vi "Main Page.vi"(8 "error in (no error)":errorcluster, 11 "Node Ptr":T1 format="%.0x") -> (0 "error out":errorcluster)   [LabVIEW 2012, in "PXImc System Explorer.lvlib"]
uses:
  PXImc System Explorer.lvlib
  <vilib>/NI Veristand/Custom Device API/Custom Device Item Ref.ctl
  Shared/Constants.vi
  <vilib>/NI Veristand/Custom Device API/Get Item Property (String).vi
  <vilib>/NI Veristand/Custom Device API/Get Item Property (U16).vi
  <vilib>/NI Veristand/Custom Device API/Set Item Property (String).vi
  <vilib>/NI Veristand/Custom Device API/Set Item Property (U16).vi
  <vilib>/NI Veristand/Custom Device API/Custom Device API.lvlib
  Shared/PXImc Shared.lvlib
panel:
  in  "Module Name":string
  in  "Remote write ID":u16
  in  "My write ID":u16
  in  "Header":cluster{"Section Name":string}={"Section Name"="PXImc Settings"}
  in  "Description":string
  in  "Name":string
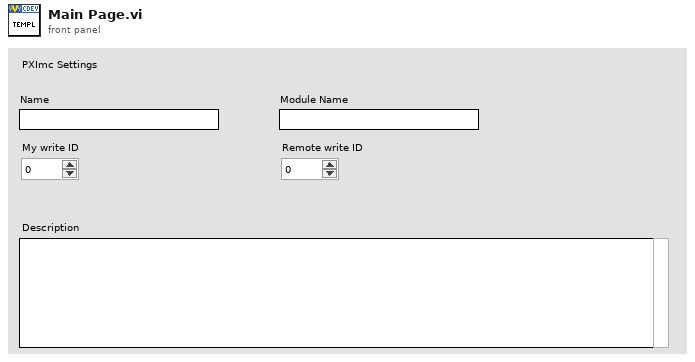
[diagram p1: front panel]
types:
  T1 = typedef "Custom Device API.lvlib/Custom Device Item Ref.ctl" = u64
  T2 = typedef "Custom Device API.lvlib/Custom Device Item Info.ctl" = cluster{"Name":string, "Is Channel":bool, "GUID":string, "Is Waveform":bool}
  T3 = typedef "Custom Device API.lvlib/Custom Device Commands.ctl" = enum16{"Default", "Item renamed", "Shutdown", "Dynamic button pressed"}
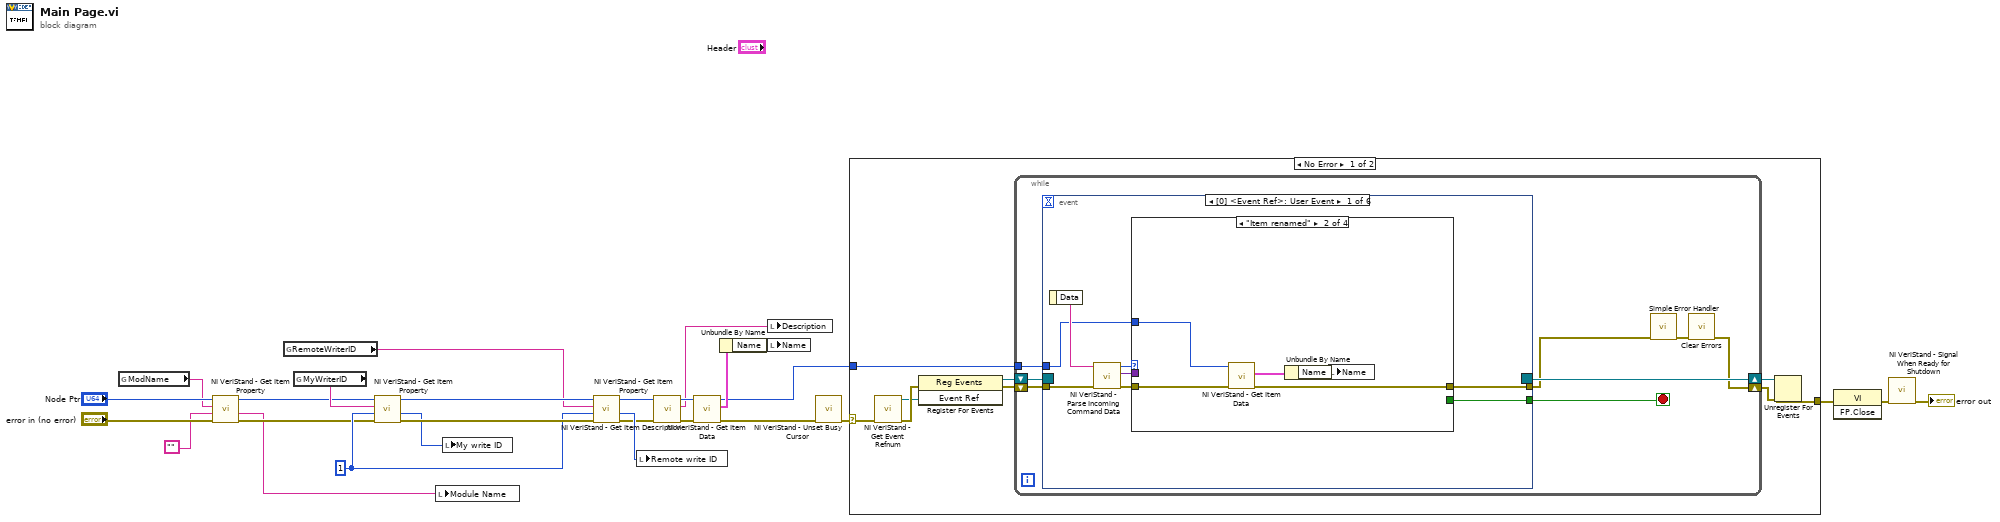
[diagram p0: block diagram]
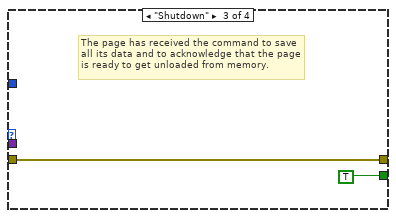
[diagram p3: hidden frame]
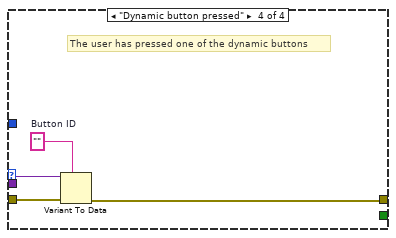
[diagram p4: hidden frame]
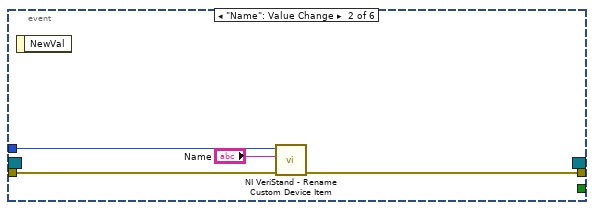
[diagram p5: hidden frame]
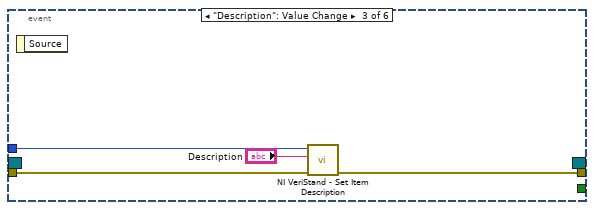
[diagram p6: hidden frame]
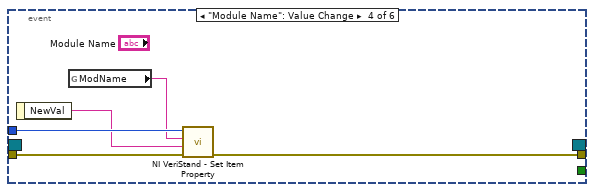
[diagram p7: hidden frame]
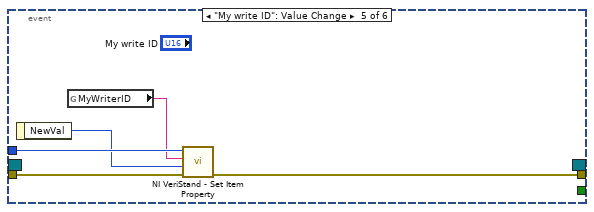
[diagram p8: hidden frame]
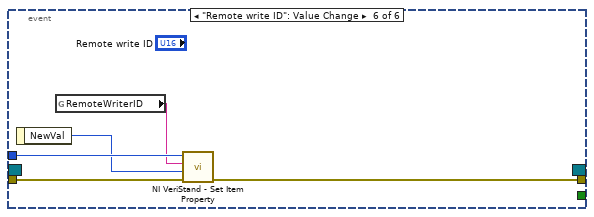
[diagram p9: hidden frame]
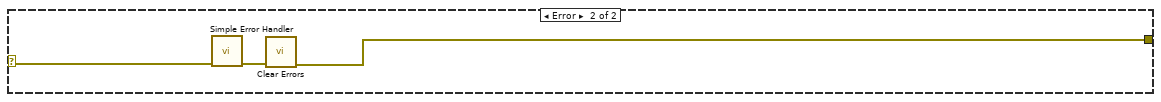
[diagram p10: hidden frame]
diagram:
  w12 = u16 1 ("Default Value")
  n1 = global read "Constants.vi" "ModName"() -> (w3:string)
  n2 = call-poly <vilib>:"NI VeriStand - Get Item Property.vi"("error in (no error)"="error in (no error)", "Default Value"="", "Property Name"=w3, "Item Ref in"="Node Ptr") -> ("error out"=w6:errorcluster, "Value"=w1:string, "Item Ref out"=w4:T1)  [unwired: 4 in, 1 out]
  n3 = global read "Constants.vi" "RemoteWriterID"() -> (w14:string)
  n4 = global read "Constants.vi" "MyWriterID"() -> (w16:string)
  n5 = call-poly <vilib>:"NI VeriStand - Get Item Property.vi"("error in (no error)"=w6, "Default Value"=w12, "Property Name"=w16, "Item Ref in"=w4) -> ("error out"=w17:errorcluster, "Value"=w13:u16, "Item Ref out"=w15:T1)  [unwired: 4 in, 1 out]
  n6 = local write "Module Name"(w1) -> ()
  n7 = local write "My write ID"(w13) -> ()
  n8 = call-poly <vilib>:"NI VeriStand - Get Item Property.vi"("error in (no error)"=w17, "Default Value"=w12, "Property Name"=w14, "Item Ref in"=w15) -> ("error out"=w9:errorcluster, "Value"=w11:u16, "Item Ref out"=w10:T1)  [unwired: 4 in, 1 out]
  n9 = local write "Remote write ID"(w11) -> ()
  n10 = call <vilib>:"NI VeriStand - Get Item Description.vi"("error in (no error)"=w9, "Item Ref in"=w10) -> ("error out"=w21:errorcluster, "Description"=w22:string, "Item Ref out"=w23:T1)  [unwired: 7 out]
  n11 = call <vilib>:"NI VeriStand - Get Item Data.vi"("error in (no error)"=w21, "Item Ref in"=w23) -> ("error out"=w8:errorcluster, "Item Info"=w20:T2, "Item Ref out"=w7:T1)  [unwired: 7 out]
  n12 = Unbundle By Name(w20) -> ("Name"=w19:string)
  n13 = local write "Description"(w22) -> ()
  n14 = local write "Name"(w19) -> ()
  n15 = call <vilib>:"NI VeriStand - Unset Busy Cursor.vi"("error in (no error)"=w8) -> ("error out"=w24:errorcluster)  [unwired: 10 out]
  n16 = case shown="No Error" w24 {
    selector: w24 -> [w29 w90]
    tunnel: [w33 w88] -> w27
    tunnel: w7 -> [w28 _]
    frame No Error {
      n17 = call <vilib>:"NI VeriStand - Get Event Refnum.vi"("error in (no error)"=w29) -> ("error out"=w36:errorcluster, "Event Ref"=w32:refnum<user-event>)  [unwired: 9 out]
      n18 = register-events(error in=w36, w32) -> (reference out=w30:refnum<event-registration>, error out=w31:errorcluster)  [unwired: 1 in]
      n19 = while {
        shift-right: [w39] -> w34
        shift-left: w31 -> [w43]
        shift-right: [w44] -> w35
        shift-left: w30 -> [w42]
        tunnel: w28 -> [w37]
        stop <- w41 stop-if-true
        n20 = event shown="[0] <Event Ref>: User Event" {
          selector: w42 -> [_ _ _ _ _ _]
          dyn-events: [_ _ _ _ _ _] -> w44
          timeout: _ -> [_ _ _ _ _ _]
          tunnel: w43 -> [w52 w68 w72 w77 w82 w87]
          tunnel: [w48 _ _ _ _ _] -> w41
          tunnel: [w47 w67 w71 w75 w80 w85] -> w38
          tunnel: w37 -> [w45 w65 w69 w76 w81 w86]
          event User Event {
            n21 = event-data() -> ("Data"=w51:string)  [unwired: 1 out]
            n22 = call <vilib>:"NI VeriStand - Parse Incoming Command Data.vi"("error in (no error)"=w52, "Incoming data"=w51) -> ("error out"=w50:errorcluster, "Outgoing data"=w46:variant, "Action"=w49:T3)  [unwired: 7 out]
            n23 = case shown="\"Item renamed\"" w49 {
              tunnel: w50 -> [w53 w58 w59 w64]
              tunnel: [_ _ TRUE _] -> w48
              tunnel: [w53 w56 w59 w61] -> w47
              tunnel: w46 -> [_ _ _ w63]
              tunnel: w45 -> [_ w54 _ _]
              frame "Default", Default {
              }
              frame "Item renamed" {
                n24 = call <vilib>:"NI VeriStand - Get Item Data.vi"("error in (no error)"=w58, "Item Ref in"=w54) -> ("error out"=w56:errorcluster, "Item Info"=w57:T2)  [unwired: 8 out]
                n25 = Unbundle By Name(w57) -> ("Name"=w55:string)
                n26 = local write "Name"(w55) -> ()
              }
              frame "Shutdown" {
                # "The page has received the command to save all its data and to acknowledge that the page is ready to get unloaded from memory."
              }
              frame "Dynamic button pressed" {
                w62 = ""  # Button ID
                # "The user has pressed one of the dynamic buttons"
                n27 = Variant To Data(error in=w64, type=w62, Variant=w63) -> (error out=w61:errorcluster)  [unwired: 1 out]
              }
            }
          }
          event "Name": Value Change {
            n28 = event-data() -> ()  [unwired: 2 out]
            n29 = call <vilib>:"NI VeriStand - Rename Custom Device Item.vi"("error in (no error)"=w68, "New Name"="Name", "Item Ref in"=w65) -> ("error out"=w67:errorcluster)  [unwired: 1 in, 7 out]
          }
          event "Description": Value Change {
            n30 = event-data() -> ()  [unwired: 2 out]
            n31 = call <vilib>:"NI VeriStand - Set Item Description.vi"("error in (no error)"=w72, "Description"="Description", "Item Ref in"=w69) -> ("error out"=w71:errorcluster)  [unwired: 8 out]
          }
          event "Module Name": Value Change {
            n32 = event-data() -> ("NewVal"=w74:string)  [unwired: 1 out]
            n33 = global read "Constants.vi" "ModName"() -> (w73:string)
            n34 = call-poly <vilib>:"NI VeriStand - Set Item Property.vi"("error in (no error)"=w77, "Value"=w74, "Property Name"=w73, "Item Ref in"=w76) -> ("error out"=w75:errorcluster)  [unwired: 5 in, 2 out]
          }
          event "My write ID": Value Change {
            n35 = event-data() -> ("NewVal"=w79:u16)  [unwired: 1 out]
            n36 = global read "Constants.vi" "MyWriterID"() -> (w78:string)
            n37 = call-poly <vilib>:"NI VeriStand - Set Item Property.vi"("error in (no error)"=w82, "Value"=w79, "Property Name"=w78, "Item Ref in"=w81) -> ("error out"=w80:errorcluster)  [unwired: 5 in, 2 out]
          }
          event "Remote write ID": Value Change {
            n38 = event-data() -> ("NewVal"=w84:u16)  [unwired: 1 out]
            n39 = global read "Constants.vi" "RemoteWriterID"() -> (w83:string)
            n40 = call-poly <vilib>:"NI VeriStand - Set Item Property.vi"("error in (no error)"=w87, "Value"=w84, "Property Name"=w83, "Item Ref in"=w86) -> ("error out"=w85:errorcluster)  [unwired: 5 in, 2 out]
          }
        }
        n41 = call <vilib>:"Simple Error Handler.vi"("error in (no error)"=w38) -> ("error out"=w40:errorcluster)  [unwired: 1 in, 7 out]
        n42 = call <vilib>:"Clear Errors.vi"("error in (no error)"=w40) -> ("error out"=w39:errorcluster)  [unwired: 6 out]
      }
      n43 = Unregister For Events(event registration refnum=w35, error in=w34) -> (error out=w33:errorcluster)
    }
    frame Error {
      n44 = call <vilib>:"Simple Error Handler.vi"("error in (no error)"=w90) -> ("error out"=w89:errorcluster)  [unwired: 1 in, 7 out]
      n45 = call <vilib>:"Clear Errors.vi"("error in (no error)"=w89) -> ("error out"=w88:errorcluster)  [unwired: 6 out]
    }
  }
  n46 = invoke class="VI" method="FP.Close"(error in=w27) -> (error out=w26:errorcluster)  [unwired: 2 in, 2 out]
  n47 = call <vilib>:"NI VeriStand - Signal When Ready for Shutdown.vi"("error in (no error)"=w26) -> ("error out"=→"error out":errorcluster)  [unwired: 10 out]
